vi "TimerEngine.GetTimeProid.vi"(8 "error in (no error)":errorcluster) -> (0 "error out":errorcluster, 3 "TimePeroid(ms)":i32)   [LabVIEW 2017, in "TimerEngine.lvlib" / "TimerEngine.lvclass"]
uses:
  TimerEngine.lvclass
  TimerEngine.lvclass/TimerEngine.ctl
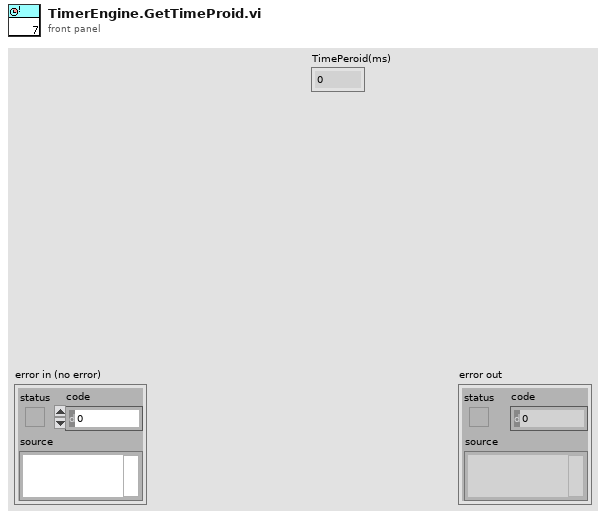
[diagram p1: front panel]
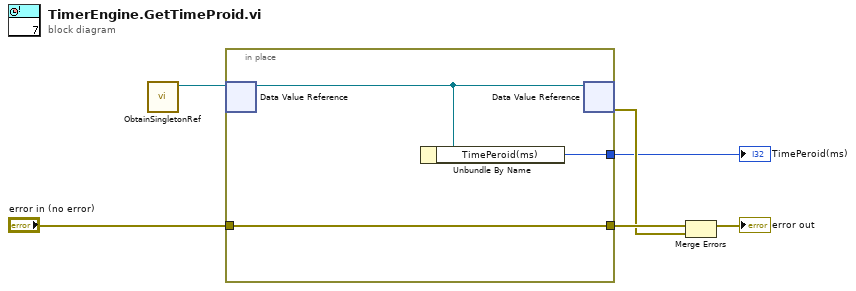
[diagram p0: block diagram]
diagram:
  n1 = call "ObtainSingletonRef.vi"() -> ("data value reference"=w6:refnum<data-value>)  [unwired: 10 in, 1 out]
  n2 = in-place {
    in-place-border: [w9] -> w5
    in-place-border: "error in (no error)" -> [w9]
    in-place-border: [w7] -> w1
    n3 = in-place-dvr #1(w6) -> (w8:refnum<class "TimerEngine.lvclass">)  [unwired: 1 out]
    n4 = Unbundle By Name(w8) -> ("TimePeroid(ms)"=w7:i32)
    n5 = in-place-dvr #1(w8) -> (w2:errorcluster)  [unwired: 1 out]
  }
  "TimePeroid(ms)" <- w1
  n6 = Merge Errors(w5, w2) -> (→"error out":errorcluster)
